vi "Get Value as Variant.vi"(8 "error in (no error)":errorcluster, 11 "CVT_Boolean in":refnum<class "CVT_Boolean.lvclass">) -> (0 "error out":errorcluster, 2 "data":variant, 3 "CVT_Boolean out":refnum<class "CVT_Boolean.lvclass">)   [LabVIEW 2024, in "Current Value Table.lvlib" / "CVT_Boolean.lvclass"]
uses:
  CVT_Boolean.lvclass
  CVT_Boolean.lvclass/CVT_Boolean.ctl
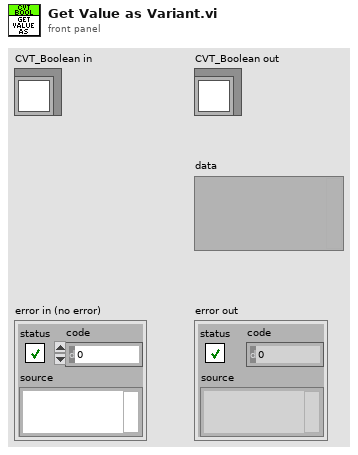
[diagram p1: front panel]
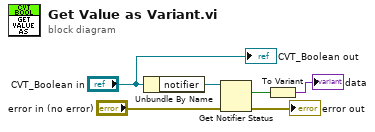
[diagram p0: block diagram]
diagram:
  n1 = Unbundle By Name("CVT_Boolean in") -> ("notifier"=w5:refnum<notifier>)
  n2 = Get Notifier Status(notifier=w5, error in (no error)="error in (no error)") -> (current notification=w4:bool, error out=→"error out":errorcluster)  [unwired: 3 out]
  n3 = To Variant(anything=w4) -> (Variant=→"data":variant)
  "CVT_Boolean out" <- "CVT_Boolean in"
